vi "Raw data save.vi"(9 "Enum":enum16{"LOCKIN", "RAW"}(ring), 10 "Input":dbl[][](array[numeric]), 11 "file format":string) -> ()   [LabVIEW 2019]
uses:
  <vilib>/Utility/file.llb/Write Delimited Spreadsheet (DBL).vi
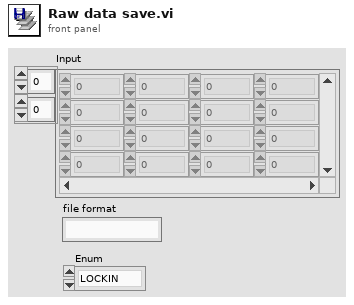
[diagram p1: front panel]
types:
  T1 = enum16{"open", "replace", "create", "open or create", "replace or create", "replace or create with confirmation"}
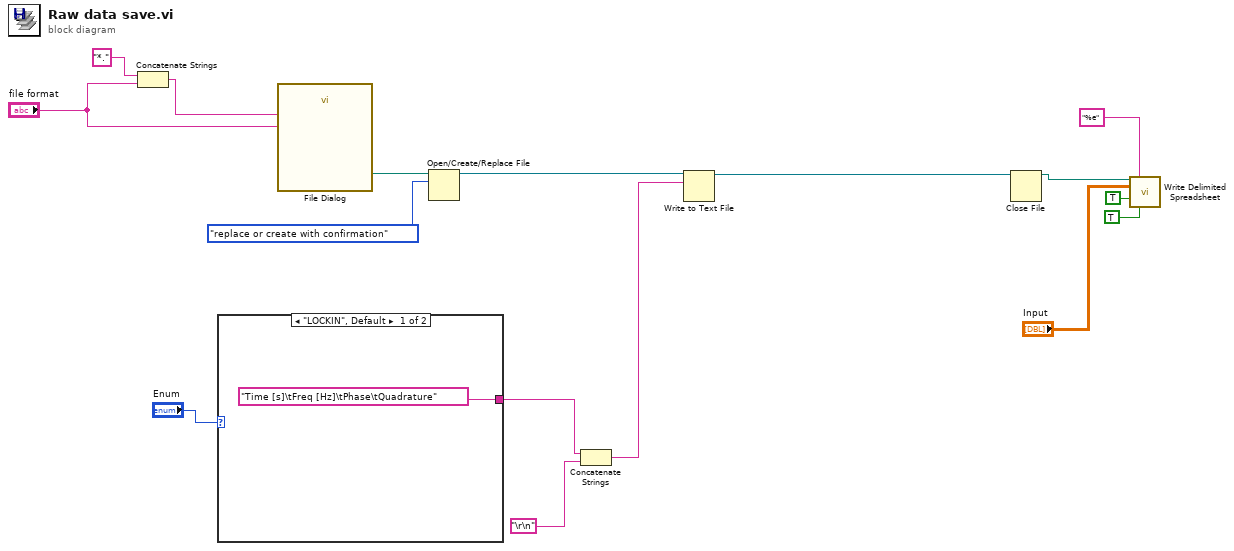
[diagram p0: block diagram]
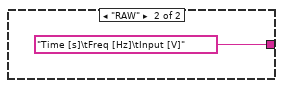
[diagram p2: hidden frame]
diagram:
  n1 = Concatenate Strings("*." ("string"), "file format") -> (w12:string)
  n2 = case shown="\"LOCKIN\", Default" "Enum" {
    tunnel: ["Time [s]\tFreq [Hz]\tPhase\tQuadrature" "Time [s]\tFreq [Hz]\tInput [V]"] -> w1
    frame "LOCKIN", Default {
    }
    frame "RAW" {
    }
  }
  n3 = call "File Dialog"("pattern (all files)"=w12, "pattern label"="file format") -> ("selected path"=w10:path)  [unwired: 10 in, 3 out]
  n4 = Open/Create/Replace File(file path (use dialog)=w10, operation (0:open)=T1."replace or create with confirmation") -> (refnum out=w8:refnum<file>)  [unwired: 4 in, 2 out]
  n5 = Concatenate Strings(w1, "\r\n") -> (w6:string)
  n6 = Write to Text File(file (use dialog)=w8, text=w6) -> (refnum out=w7:refnum<file>)  [unwired: 2 in, 2 out]
  n7 = Close File(refnum=w7) -> (path=w9:path)  [unwired: 1 in, 1 out]
  n8 = call-poly <vilib>:"Write Delimited Spreadsheet.vi"("file path (dialog if empty)"=w9, "format (%.3f)"="%e", "2D data"="Input", "append to file? (new file:F)"=TRUE, "transpose? (no:F)"=TRUE) -> ()  [unwired: 9 in, 2 out]
